vi "Process.vi"(8 "error in":errorcluster, 11 "DAQmx":refnum<class "DAQmx.lvclass">) -> (0 "error out":errorcluster, 3 "DAQmx out":refnum<class "DAQmx.lvclass">)   [LabVIEW 2019, in "DAQmx.lvclass"]
uses:
  DAQmx.lvclass
  C:/Program Files/National Instruments/LabVIEW 2019/vi.lib/JKI/JKI SMO/SMO/SMO.lvclass
  typedefs/DAQmx.Status--enum.ctl
  typedefs/DAQmx.Commands--enum.ctl
  <vilib>/JKI/JKI SMO/SMO/SMO.lvclass/SMO.ctl
  DAQmx.lvclass/DAQmx.ctl
  typedefs/Message--Cluster.ctl
  typedefs/DAQ.Config.Timing--Cluster.ctl
  typedefs/DAQ.Config.Timing.Sampling--Cluster.ctl
  typedefs/DAQ.Config.Timing.Fs Mode--enum.ctl
  <userlib>/LevyLab/Debug/Attribute.Debug/DebugBehavior.ctl
  45607b6f-cbbd-4354-99c2-ae126d9fef0d.vi
  <vilib>/JKI/JKI SMO/SMO/Private/ReftoDVR--SMO.vi
  <vilib>/JKI/JKI SMO/SMO/SMO.lvclass
  <userlib>/LevyLab/Debug/Debug.lvlib
  <userlib>/LevyLab/Debug/Attribute.Debug/Attribute.Debug.lvclass
panel:
  out "Error":string
  out "event loop":i32
  out "acq loop":i32
  out "Command":T1
  out "Status":T2
  out "State":string
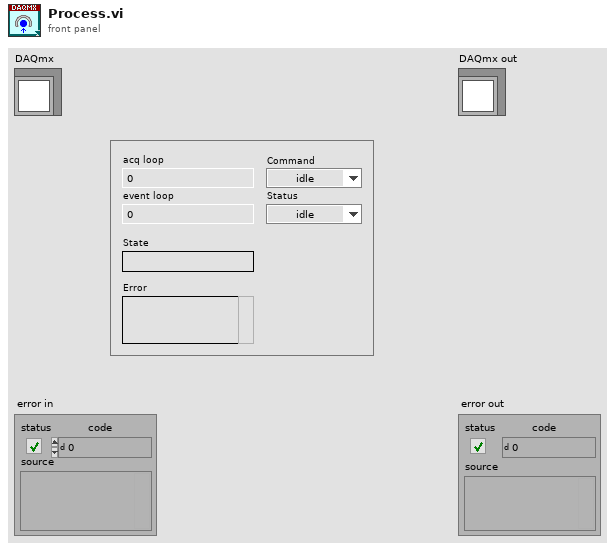
[diagram p1: front panel]
types:
  T1 = typedef "DAQmx.lvclass/DAQmx.Commands--enum.ctl" = enum16{"idle", "start", "stop", "calibrate", "auto", "exit"}
  T2 = typedef "DAQmx.lvclass/DAQmx.Status--enum.ctl" = enum16{"idle", "calibrating", "configuring", "creating", "created", "starting", "started", "stopping", "stopped", "clearing", "error"}
  T3 = typedef "Debug.lvlib/Attribute.Debug.lvclass/DebugBehavior.ctl" = enum16{"Normal", "Debug"}
  T4 = enum32{"Invalid", "Standard", "Closed", "Hidden", "Minimized", "Maximized"}
  T5 = typedef "DAQmx.lvclass/Message--Cluster.ctl" = cluster{"command":T1, "Argument":string}
  T6 = typedef "DAQmx.lvclass/DAQ.Config.Timing--Cluster.ctl" = cluster{"Sampling":T7, "sample mode":i32, "FsMode":T8, "Fs Multiplier":dbl, "Refresh Rate (Hz)":dbl, "Decimation.PreDSP":i32, "Decimation.PostDSP":i32, "Fs.Output":dbl}
  T7 = typedef "DAQmx.lvclass/DAQ.Config.Timing.Sampling--Cluster.ctl" = cluster{"Fs":dbl, "#s":i32}
  T8 = typedef "DAQmx.lvclass/DAQ.Config.Timing.Fs Mode--enum.ctl" = enum16{"Manual", "Auto Fs", "Max Fs"}
  T9 = typedef "SMO.lvclass/Protected Events.ctl" = cluster{"StopProcesses":refnum<user-event>, "AbortProcesses":refnum<user-event>, "Config Changed":refnum<user-event>, "Dependency":refnum<user-event>}
  T10 = typedef "DAQmx.lvclass/PrivateEvents--Cluster.ctl" = cluster{"Message":refnum<user-event>, "AOconfig":refnum<user-event>, "AIconfig":refnum<user-event>, "Timing":refnum<user-event>}
  T11 = cluster{"Active Device":string, "SelfCal.LastDate/Time":string, "SelfCal.LastTemp":dbl, "DevTemp":dbl, "calibration due?":bool}[]
  T12 = typedef "DAQmx.lvclass/DeviceInfo--Cluster.ctl" = cluster{"DeviceName":string, "DevIsSimulated":bool, "DeviceSerialNumber":string, "ProductType":string, "ProductCategory":i32, "ProductNumber":u32, "ChassisNumber":u32, "SlotNumber":u32, "ChassisName":string, "ChassisSerialNumber":string, "DevTemp":dbl, "SelfCal.LastDate/Time":string, "SelfCal.LastTemp":dbl, "calibration due?":bool}
  T13 = typedef "DAQmx.lvclass/DAQ.Config.AI--Cluster--Array.ctl" = T14[]
  T14 = typedef "DAQmx.lvclass/DAQ.Config.AI--Cluster.ctl" = cluster{"Channels":tag, "Coupling":T15, "Range":T16, "input terminal configuration":i32, "Type":T17}
  T15 = typedef "DAQmx.lvclass/DAQ.Config.AI.Coupling--enum.ctl" = u16
  T16 = typedef "DAQmx.lvclass/DAQ.Config.AI.Range--enum.ctl" = enum16{"±0.316", "±1.00", "±3.16", "±10.0", "±31.6", "±42.4", ""}
  T17 = typedef "DAQmx.lvclass/DAQ.Config.Device Type--enum.ctl" = enum16{"None", "USB-4431", "PXI-446x"}
  T18 = typedef "DAQmx.lvclass/DAQ.Config.AO--Cluster--Array.ctl" = T19[]
  T19 = typedef "DAQmx.lvclass/DAQ.Config.AO--Cluster.ctl" = cluster{"Channels":tag, "Range":T20, "output terminal configuration":i32, "Type":T17}
  T20 = typedef "DAQmx.lvclass/DAQ.Config.AO.Range--enum.ctl" = enum16{"±0.1", "±1.0", "±3.5", "±10.0", ""}
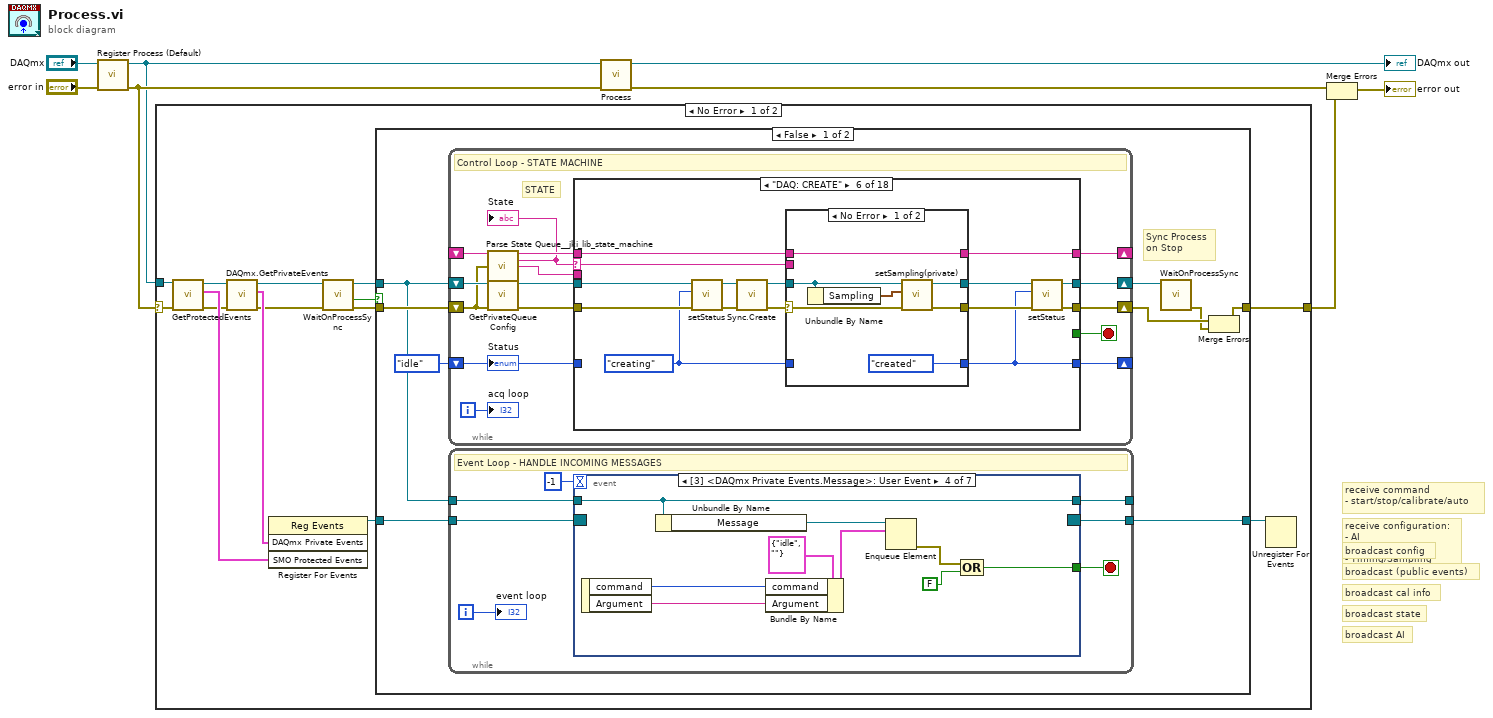
[diagram p0: block diagram]
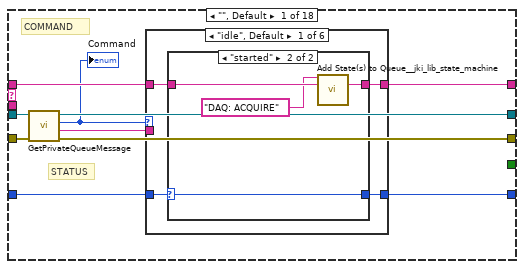
[diagram p2: hidden frame]
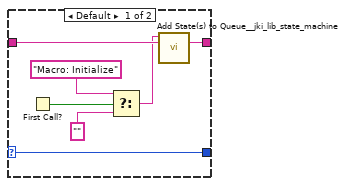
[diagram p3: hidden frame]
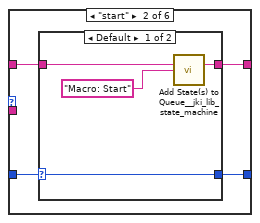
[diagram p4: hidden frame]
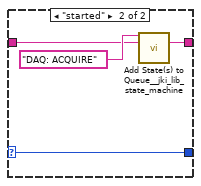
[diagram p5: hidden frame]
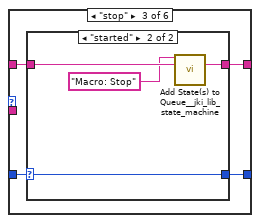
[diagram p6: hidden frame]
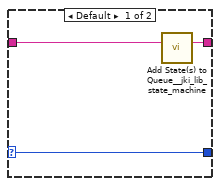
[diagram p7: hidden frame]
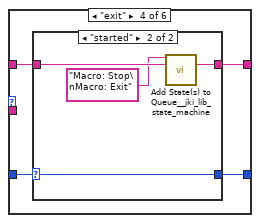
[diagram p8: hidden frame]
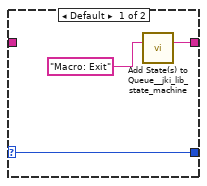
[diagram p9: hidden frame]
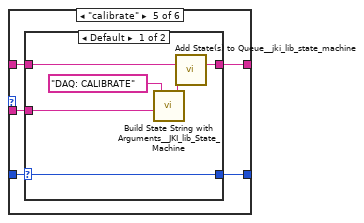
[diagram p10: hidden frame]
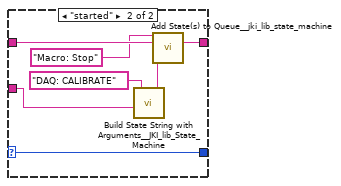
[diagram p11: hidden frame]
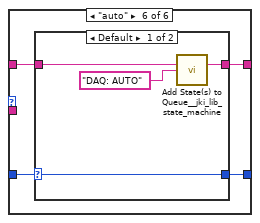
[diagram p12: hidden frame]
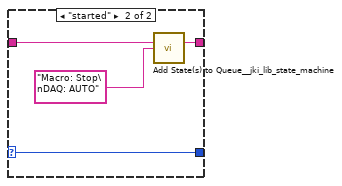
[diagram p13: hidden frame]
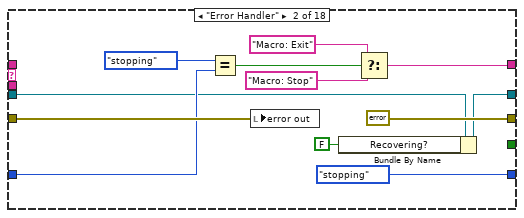
[diagram p14: hidden frame]
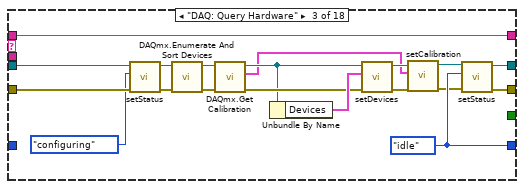
[diagram p15: hidden frame]
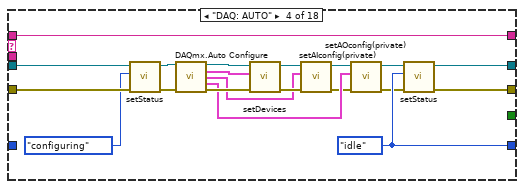
[diagram p16: hidden frame]
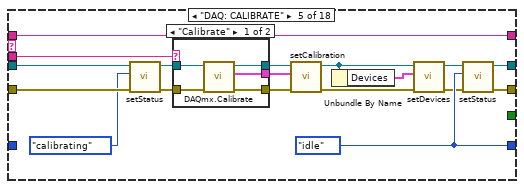
[diagram p17: hidden frame]
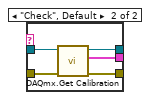
[diagram p18: hidden frame]
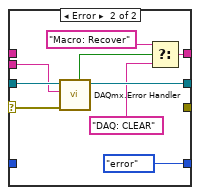
[diagram p19: hidden frame]
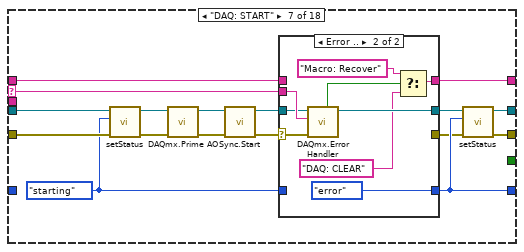
[diagram p20: hidden frame]
diagram:
  # "broadcast (public events)"
  # "receive configuration:\n- AI\n- AO\n- Timing/Sampling"
  # "receive command\n- start/stop/calibrate/auto"
  # "broadcast AI"
  # "broadcast state"
  # "broadcast cal info"
  # "broadcast config"
  n1 = call <vilib>:"Register Process (Default).vi"("error in (no error)"="error in", "SMO"="DAQmx") -> ("error out"=w3:errorcluster, "SelfRef"=w1:refnum<class "DAQmx.lvclass">)  [unwired: 8 in]
  n2 = case shown="No Error" w3 {
    selector: w3 -> [w20 w555]
    tunnel: w1 -> [w21 _]
    tunnel: [w16 w555] -> w8
    frame No Error {
      n3 = call <vilib>:"GetProtectedEvents.vi"("error in (no error)"=w20, "SMO"=w21) -> ("error out"=w13:errorcluster, "SMO Protected Events"=w22:T9, "SMO out"=w12:refnum<class "DAQmx.lvclass">)  [unwired: 7 in]
      n4 = call "DAQmx.GetPrivateEvents.vi"("error in (no error)"=w13, "DAQmx"=w12) -> ("error out"=w9:errorcluster, "DAQmx Private Events"=w11:T10, "DAQmx out"=w10:refnum<class "DAQmx.lvclass">)  [unwired: 7 in]
      n5 = register-events(w11, w22) -> (reference out=w14:refnum<event-registration>)  [unwired: 2 in, 1 out]
      n6 = call <vilib>:"WaitOnProcessSync.vi"("error in (no error)"=w9, "SMO"=w10) -> ("error out"=w18:errorcluster, "Don't run?"=w17:bool, "SMO out"=w19:refnum<class "DAQmx.lvclass">)  [unwired: 7 in]
      n7 = case shown="False" w17 {
        tunnel: w18 -> [w28 w553]
        tunnel: w19 -> [w23 _]
        tunnel: w14 -> [w30 w554]
        tunnel: [w25 w553] -> w16
        tunnel: [w29 w554] -> w15
        frame False {
          # "Sync Process\non Stop"
          n8 = while {
            shift-right: [w44] -> w31
            shift-left: w23 -> [w39]
            shift-right: [w36] -> w27
            shift-left: w28 -> [w33]
            shift-right: [w43] -> _
            shift-left: _ -> [w46]
            shift-right: [w45] -> _
            shift-left: DAQmx.Status--enum."idle" ("Status") -> [w40]
            i -> [w34]
            stop <- w32 stop-if-true
            # "STATE"
            # "Control Loop - STATE MACHINE"
            n9 = call <vilib>:"Parse State Queue__jki_lib_state_machine.vi"("State Queue"=w46, "Error In (no error)"=w33) -> ("Remaining States"=w42:string, "Current State"=w41:string, "Arguments"=w35:string)  [unwired: 11 in]
            "State" <- w41
            n10 = call "GetPrivateQueueConfig.vi"("error in (no error)"=w33, "DAQmx"=w39) -> ("error out"=w37:errorcluster, "DAQmx out"=w38:refnum<class "DAQmx.lvclass">)  [unwired: 8 in]
            n11 = case shown="\"DAQ: CREATE\"" w41 {
              selector: w41 -> [_ _ _ _ _ w222 w252 w287 w325 w348 _ _ _ _ _ _ _ _]
              tunnel: w38 -> [w51 w137 w158 w180 w202 w228 w261 w293 w330 w353 w368 w371 w377 w391 w401 w421 w431 w495]
              tunnel: [w52 w136 w159 w175 w195 w216 w248 w284 w323 w344 w368 w371 w378 w392 w399 w415 w431 w497] -> w44
              tunnel: [w49 errorcluster {"status"=FALSE, "code"=0, "source"=""} ("error out") w160 w174 w196 w215 w247 w285 w322 w345 w367 w372 w381 w390 w398 w424 _ w496] -> w36
              tunnel: w37 -> [w50 w141 w163 w179 w201 w229 w260 w292 w331 w357 w367 w372 w381 w389 w400 w420 _ w494]
              tunnel: w35 -> [_ _ _ _ w204 _ _ _ _ _ _ _ _ _ _ _ w428 _]
              tunnel: w42 -> [w53 _ w166 w186 w194 w220 w253 w290 w326 w350 _ w374 w383 w393 w409 w423 w430 w493]
              tunnel: [w56 w139 w166 w186 w194 w221 w254 w291 w327 w349 "UI: Initialize\nDAQ: Query Hardware" ("States Out") w375 w384 w394 w410 w427 w430 w493] -> w43
              tunnel: [w54 DAQmx.Status--enum."stopping" ("Status") w161 w178 w197 w217 w251 w286 w320 w343 w366 w370 w380 w395 w408 w426 w432 w499] -> w45
              tunnel: w40 -> [w55 w140 _ _ _ _ _ w289 _ _ w366 w370 w380 w395 w408 w426 w432 w499]
              tunnel: [_ _ _ _ _ _ _ _ _ _ _ _ _ _ _ _ _ TRUE] -> w32
              frame "", Default {
                # "STATUS"
                # "COMMAND"
                n12 = call "GetPrivateQueueMessage.vi"("error in (no error)"=w50, "DAQmx"=w51) -> ("error out"=w49:errorcluster, "argument"=w47:string, "command"=w48:T1, "DAQmx out"=w52:refnum<class "DAQmx.lvclass">)  [unwired: 6 in]
                "Command" <- w48
                n13 = case shown="\"idle\", Default" w48 {
                  tunnel: w55 -> [w60 w75 w87 w98 w110 w127]
                  tunnel: [w58 w74 w86 w97 w109 w126] -> w56
                  tunnel: [w59 w73 w85 w96 w108 w125] -> w54
                  tunnel: w53 -> [w57 w72 w84 w95 w107 w124]
                  tunnel: w47 -> [_ _ _ _ w106 _]
                  frame "idle", Default {
                    n14 = case shown="\"started\"" w60 {
                      selector: w60 -> [w67 w71]
                      tunnel: [w63 w69] -> w58
                      tunnel: [w67 w71] -> w59
                      tunnel: w57 -> [w62 w70]
                      frame Default {
                        n15 = First Call?() -> (First Call?: T/F=w65:bool)
                        n16 = Select(t="Macro: Initialize" ("States Out"), s=w65, f="" ("States Out")) -> (s? t:f=w61:string)
                        n17 = call <vilib>:"Add State(s) to Queue__jki_lib_state_machine.vi"("State(s) in Front (\"\")"=w61, "State(s) in (\"\")"=w62) -> ("States Out"=w63:string)  [unwired: 13 in]
                      }
                      frame "started" {
                        n18 = call <vilib>:"Add State(s) to Queue__jki_lib_state_machine.vi"("State(s) in Front (\"\")"="DAQ: ACQUIRE" ("State(s) in (\"\")"), "State(s) in (\"\")"=w70) -> ("States Out"=w69:string)  [unwired: 13 in]
                      }
                    }
                  }
                  frame "start" {
                    n19 = case shown="Default" w75 {
                      selector: w75 -> [w79 w83]
                      tunnel: [w77 w82] -> w74
                      tunnel: [w79 w83] -> w73
                      tunnel: w72 -> [w78 w80]
                      frame Default {
                        n20 = call <vilib>:"Add State(s) to Queue__jki_lib_state_machine.vi"("State(s) in (\"\")"=w78, "State(s) at Back (\"\")"="Macro: Start" ("State(s) in (\"\")")) -> ("States Out"=w77:string)  [unwired: 13 in]
                      }
                      frame "started" {
                        n21 = call <vilib>:"Add State(s) to Queue__jki_lib_state_machine.vi"("State(s) in Front (\"\")"="DAQ: ACQUIRE" ("State(s) in (\"\")"), "State(s) in (\"\")"=w80) -> ("States Out"=w82:string)  [unwired: 13 in]
                      }
                    }
                  }
                  frame "stop" {
                    n22 = case shown="\"started\"" w87 {
                      selector: w87 -> [w90 w94]
                      tunnel: [w88 w92] -> w86
                      tunnel: [w90 w94] -> w85
                      tunnel: w84 -> [w89 w93]
                      frame Default {
                        n23 = call <vilib>:"Add State(s) to Queue__jki_lib_state_machine.vi"("State(s) in (\"\")"=w89) -> ("States Out"=w88:string)  [unwired: 14 in]
                      }
                      frame "started" {
                        n24 = call <vilib>:"Add State(s) to Queue__jki_lib_state_machine.vi"("State(s) in Front (\"\")"="Macro: Stop" ("State(s) in (\"\")"), "State(s) in (\"\")"=w93) -> ("States Out"=w92:string)  [unwired: 13 in]
                      }
                    }
                  }
                  frame "exit" {
                    n25 = case shown="\"started\"" w98 {
                      selector: w98 -> [w101 w105]
                      tunnel: [w100 w102] -> w97
                      tunnel: [w101 w105] -> w96
                      tunnel: w95 -> [_ w104]
                      frame Default {
                        n26 = call <vilib>:"Add State(s) to Queue__jki_lib_state_machine.vi"("State(s) in (\"\")"="Macro: Exit" ("State(s) in (\"\")")) -> ("States Out"=w100:string)  [unwired: 14 in]
                      }
                      frame "started" {
                        n27 = call <vilib>:"Add State(s) to Queue__jki_lib_state_machine.vi"("State(s) in Front (\"\")"="Macro: Stop\nMacro: Exit" ("State(s) in (\"\")"), "State(s) in (\"\")"=w104) -> ("States Out"=w102:string)  [unwired: 13 in]
                      }
                    }
                  }
                  frame "calibrate" {
                    n28 = case shown="Default" w110 {
                      selector: w110 -> [w116 w123]
                      tunnel: [w114 w121] -> w109
                      tunnel: [w116 w123] -> w108
                      tunnel: w107 -> [w115 w122]
                      tunnel: w106 -> [w113 w119]
                      frame Default {
                        n29 = call <vilib>:"Build State String with Arguments__JKI_lib_State_Machine.vi"("Arguments (\"\")"=w113, "State"="DAQ: CALIBRATE" ("State(s) in (\"\")")) -> ("State with Arguments"=w111:string)  [unwired: 4 in]
                        n30 = call <vilib>:"Add State(s) to Queue__jki_lib_state_machine.vi"("State(s) in (\"\")"=w115, "State(s) at Back (\"\")"=w111) -> ("States Out"=w114:string)  [unwired: 13 in]
                      }
                      frame "started" {
                        n31 = call <vilib>:"Build State String with Arguments__JKI_lib_State_Machine.vi"("Arguments (\"\")"=w119, "State"="DAQ: CALIBRATE" ("State(s) in (\"\")")) -> ("State with Arguments"=w117:string)  [unwired: 4 in]
                        n32 = call <vilib>:"Add State(s) to Queue__jki_lib_state_machine.vi"("State(s) in Front (\"\")"="Macro: Stop" ("State(s) in (\"\")"), "State(s) in (\"\")"=w122, "State(s) at Back (\"\")"=w117) -> ("States Out"=w121:string)  [unwired: 12 in]
                      }
                    }
                  }
                  frame "auto" {
                    n33 = case shown="Default" w127 {
                      selector: w127 -> [w131 w135]
                      tunnel: [w129 w133] -> w126
                      tunnel: [w131 w135] -> w125
                      tunnel: w124 -> [w130 w134]
                      frame Default {
                        n34 = call <vilib>:"Add State(s) to Queue__jki_lib_state_machine.vi"("State(s) in (\"\")"=w130, "State(s) at Back (\"\")"="DAQ: AUTO" ("State(s) in (\"\")")) -> ("States Out"=w129:string)  [unwired: 13 in]
                      }
                      frame "started" {
                        n35 = call <vilib>:"Add State(s) to Queue__jki_lib_state_machine.vi"("State(s) in (\"\")"=w134, "State(s) at Back (\"\")"="Macro: Stop\nDAQ: AUTO" ("State(s) in (\"\")")) -> ("States Out"=w133:string)  [unwired: 13 in]
                      }
                    }
                  }
                }
              }
              frame "Error Handler" {
                n36 = Equal?(x=DAQmx.Status--enum."stopping" ("Status"), y=w140) -> (x = y?=w143:bool)
                n37 = local write "error out"(w141) -> ()
                n38 = Bundle By Name(cluster=w137, "Recovering?"=FALSE ("Recovery.Recovering?")) -> (w136:refnum<class "DAQmx.lvclass">)
                n39 = Select(t="Macro: Exit", s=w143, f="Macro: Stop" ("States Out")) -> (s? t:f=w139:string)
              }
              frame "DAQ: Query Hardware" {
                w161 = DAQmx.Status--enum."idle" ("setStatus")
                n40 = call "setStatus.vi"("error in (no error)"=w163, "Status"=DAQmx.Status--enum."configuring" ("setStatus"), "DAQmx in"=w158) -> ("error out"=w164:errorcluster, "DAQmx out"=w165:refnum<class "DAQmx.lvclass">)  [unwired: 7 in]
                n41 = call "DAQmx.Enumerate And Sort Devices.vi"("error in (no error)"=w164, "DAQmx in"=w165) -> ("error out"=w157:errorcluster, "DAQmx out"=w156:refnum<class "DAQmx.lvclass">)  [unwired: 7 in, 1 out]
                n42 = call "DAQmx.Get Calibration.vi"("error in (no error)"=w157, "DAQmx in"=w156) -> ("error out"=w154:errorcluster, "Calibration out"=w148:T11, "DAQmx out"=w153:refnum<class "DAQmx.lvclass">)  [unwired: 7 in]
                n43 = Unbundle By Name(w153) -> ("Devices"=w155:T12[])
                n44 = call "setDevices.vi"("error in (no error)"=w154, "Devices"=w155, "DAQmx in"=w153) -> ("error out"=w152:errorcluster, "DAQmx out"=w151:refnum<class "DAQmx.lvclass">)  [unwired: 7 in]
                n45 = call "setCalibration.vi"("error in (no error)"=w152, "Calibration out"=w148, "DAQmx in"=w151) -> ("error out"=w149:errorcluster, "DAQmx out"=w150:refnum<class "DAQmx.lvclass">)  [unwired: 7 in]
                n46 = call "setStatus.vi"("error in (no error)"=w149, "Status"=w161, "DAQmx in"=w150) -> ("error out"=w160:errorcluster, "DAQmx out"=w159:refnum<class "DAQmx.lvclass">)  [unwired: 7 in]
              }
              frame "DAQ: AUTO" {
                w178 = DAQmx.Status--enum."idle" ("setStatus")
                n47 = call "setStatus.vi"("error in (no error)"=w179, "Status"=DAQmx.Status--enum."configuring" ("setStatus"), "DAQmx in"=w180) -> ("error out"=w182:errorcluster, "DAQmx out"=w181:refnum<class "DAQmx.lvclass">)  [unwired: 7 in]
                n48 = call "DAQmx.Auto Configure.vi"("DAQmx in"=w181, "error in (no error)"=w182) -> ("DAQmx out"=w184:refnum<class "DAQmx.lvclass">, "Devices"=w167:T12[], "Configuration.AI"=w169:T13, "Configuration.AO"=w177:T18, "error out"=w185:errorcluster)  [unwired: 9 in]
                n49 = call "setDevices.vi"("error in (no error)"=w185, "Devices"=w167, "DAQmx in"=w184) -> ("error out"=w183:errorcluster, "DAQmx out"=w176:refnum<class "DAQmx.lvclass">)  [unwired: 7 in]
                n50 = call "setAIconfig(private).vi"("error in (no error)"=w183, "AIconfig"=w169, "DAQmx in"=w176) -> ("error out"=w172:errorcluster, "DAQmx out"=w173:refnum<class "DAQmx.lvclass">)  [unwired: 7 in]
                n51 = call "setAOconfig(private).vi"("error in (no error)"=w172, "AOconfig"=w177, "DAQmx in"=w173) -> ("error out"=w170:errorcluster, "DAQmx out"=w171:refnum<class "DAQmx.lvclass">)  [unwired: 7 in]
                n52 = call "setStatus.vi"("error in (no error)"=w170, "Status"=w178, "DAQmx in"=w171) -> ("error out"=w174:errorcluster, "DAQmx out"=w175:refnum<class "DAQmx.lvclass">)  [unwired: 7 in]
              }
              frame "DAQ: CALIBRATE" {
                w197 = DAQmx.Status--enum."idle" ("Status")
                n53 = call "setStatus.vi"("error in (no error)"=w201, "Status"=DAQmx.Status--enum."calibrating" ("setStatus"), "DAQmx in"=w202) -> ("error out"=w199:errorcluster, "DAQmx out"=w198:refnum<class "DAQmx.lvclass">)  [unwired: 7 in]
                n54 = case shown="\"Calibrate\"" w204 {
                  tunnel: w198 -> [w209 w214]
                  tunnel: [w208 w213] -> w188
                  tunnel: [w206 w212] -> w203
                  tunnel: w199 -> [w207 w211]
                  tunnel: [w205 w210] -> w193
                  frame "Calibrate" {
                    n55 = call "DAQmx.Calibrate.vi"("error in (no error)"=w207, "DAQmx in"=w209) -> ("error out"=w206:errorcluster, "Calibration out"=w205:T11, "DAQmx out"=w208:refnum<class "DAQmx.lvclass">)  [unwired: 7 in]
                  }
                  frame "Check", Default {
                    n56 = call "DAQmx.Get Calibration.vi"("error in (no error)"=w211, "DAQmx in"=w214) -> ("error out"=w212:errorcluster, "Calibration out"=w210:T11, "DAQmx out"=w213:refnum<class "DAQmx.lvclass">)  [unwired: 7 in]
                  }
                }
                n57 = call "setCalibration.vi"("error in (no error)"=w203, "Calibration out"=w193, "DAQmx in"=w188) -> ("error out"=w191:errorcluster, "DAQmx out"=w187:refnum<class "DAQmx.lvclass">)  [unwired: 7 in]
                n58 = Unbundle By Name(w187) -> ("Devices"=w192:T12[])
                n59 = call "setDevices.vi"("error in (no error)"=w191, "Devices"=w192, "DAQmx in"=w187) -> ("error out"=w189:errorcluster, "DAQmx out"=w190:refnum<class "DAQmx.lvclass">)  [unwired: 7 in]
                n60 = call "setStatus.vi"("error in (no error)"=w189, "Status"=w197, "DAQmx in"=w190) -> ("error out"=w196:errorcluster, "DAQmx out"=w195:refnum<class "DAQmx.lvclass">)  [unwired: 7 in]
              }
              frame "DAQ: CREATE" {
                w223 = DAQmx.Status--enum."creating" ("Status")
                n61 = call "setStatus.vi"("error in (no error)"=w229, "Status"=w223, "DAQmx in"=w228) -> ("error out"=w226:errorcluster, "DAQmx out"=w227:refnum<class "DAQmx.lvclass">)  [unwired: 7 in]
                n62 = call "Sync.Create.vi"("error in"=w226, "DAQmx in"=w227) -> ("error out"=w224:errorcluster, "DAQmx out"=w225:refnum<class "DAQmx.lvclass">)  [unwired: 8 in]
                n63 = case shown="No Error" w224 {
                  selector: w224 -> [w234 w244]
                  tunnel: w225 -> [w231 w245]
                  tunnel: [w233 _] -> w218
                  tunnel: [w232 w242] -> w219
                  tunnel: [DAQmx.Status--enum."created" ("Status") DAQmx.Status--enum."error" ("Status")] -> w217
                  tunnel: w223 -> [_ _]
                  tunnel: w222 -> [_ w241]
                  tunnel: [w236 w237] -> w221
                  tunnel: w220 -> [w236 _]
                  frame No Error {
                    n64 = Unbundle By Name(w231) -> ("Sampling"=w230:T7)
                    n65 = call "setSampling(private).vi"("error in (no error)"=w234, "Sampling"=w230, "DAQmx in"=w231) -> ("error out"=w233:errorcluster, "DAQmx out"=w232:refnum<class "DAQmx.lvclass">)  [unwired: 7 in]
                  }
                  frame Error {
                    n66 = call "DAQmx.Error Handler.vi"("error in (no error)"=w244, "[error source] (\" \")"=w241, "DAQmx in"=w245) -> ("DAQmx out"=w242:refnum<class "DAQmx.lvclass">, "retry?"=w240:bool)  [unwired: 4 in, 3 out]
                    n67 = Select(t="Macro: Recover", s=w240, f="DAQ: CLEAR" ("t")) -> (s? t:f=w237:string)
                  }
                }
                n68 = call "setStatus.vi"("error in (no error)"=w218, "Status"=w217, "DAQmx in"=w219) -> ("error out"=w215:errorcluster, "DAQmx out"=w216:refnum<class "DAQmx.lvclass">)  [unwired: 7 in]
              }
              frame "DAQ: START" {
                w255 = DAQmx.Status--enum."starting" ("Status")
                n69 = call "setStatus.vi"("error in (no error)"=w260, "Status"=w255, "DAQmx in"=w261) -> ("error out"=w259:errorcluster, "DAQmx out"=w257:refnum<class "DAQmx.lvclass">)  [unwired: 7 in]
                n70 = call "DAQmx.Prime AO.vi"("error in (no error)"=w259, "DAQmx in"=w257) -> ("error out"=w258:errorcluster, "DAQmx out"=w246:refnum<class "DAQmx.lvclass">)  [unwired: 8 in]
                n71 = call "Sync.Start.vi"("error in"=w258, "DAQmx in"=w246) -> ("error out"=w256:errorcluster, "DAQmx out"=w262:refnum<class "DAQmx.lvclass">)  [unwired: 8 in]
                n72 = case shown="Error .." w256 {
                  selector: w256 -> [w263 w273]
                  tunnel: w262 -> [w264 w274]
                  tunnel: [w263 _] -> w249
                  tunnel: [w264 w272] -> w250
                  tunnel: [DAQmx.Status--enum."started" ("Status") DAQmx.Status--enum."error" ("Status")] -> w251
                  tunnel: w255 -> [_ _]
                  tunnel: [w266 w270] -> w254
                  tunnel: w253 -> [w266 _]
                  tunnel: w252 -> [_ w275]
                  frame No Error {
                  }
                  frame Error {
                    n73 = call "DAQmx.Error Handler.vi"("error in (no error)"=w273, "[error source] (\" \")"=w275, "DAQmx in"=w274) -> ("DAQmx out"=w272:refnum<class "DAQmx.lvclass">, "retry?"=w269:bool)  [unwired: 4 in, 3 out]
                    n74 = Select(t="Macro: Recover", s=w269, f="DAQ: CLEAR" ("t")) -> (s? t:f=w270:string)
                  }
                }
                n75 = call "setStatus.vi"("error in (no error)"=w249, "Status"=w251, "DAQmx in"=w250) -> ("error out"=w247:errorcluster, "DAQmx out"=w248:refnum<class "DAQmx.lvclass">)  [unwired: 7 in]
              }
              frame "DAQ: ACQUIRE" {
                n76 = call "getWFMQueue.vi"("error in (no error)"=w292, "wait for min buffer?"=FALSE, "DAQmx in"=w293) -> ("error out"=w282:errorcluster, "DAQmx out"=w283:refnum<class "DAQmx.lvclass">)  [unwired: 6 in, 1 out]
                n77 = call "Sync.Acquire.vi"("error in (no error)"=w282, "DAQmx in"=w283) -> ("error out"=w281:errorcluster, "DAQmx out"=w280:refnum<class "DAQmx.lvclass">)  [unwired: 8 in]
                n78 = call "setWaveforms.vi"("error in (no error)"=w281, "DAQmx in"=w280) -> ("error out"=w278:errorcluster, "DAQmx out"=w279:refnum<class "DAQmx.lvclass">)  [unwired: 8 in]
                n79 = call "Scope.vi"("error in (no error)"=w278, "DAQmx in"=w279) -> ("error out"=w277:errorcluster, "DAQmx out"=w276:refnum<class "DAQmx.lvclass">)  [unwired: 8 in]
                n80 = case shown="Error .." w277 {
                  selector: w277 -> [_ w311]
                  tunnel: [w301 w315] -> w291
                  tunnel: w276 -> [w298 w319]
                  tunnel: [w296 w317] -> w284
                  tunnel: w290 -> [w301 _]
                  tunnel: w289 -> [w300 _]
                  tunnel: w287 -> [_ w312]
                  tunnel: [w300 w313] -> w286
                  tunnel: [w295 w318] -> w285
                  frame No Error {
                    n81 = call "Is Value Changed.vim"("value"=w300) -> ("changed or first call?"=w299:bool)
                    n82 = case shown="True" w299 {
                      tunnel: w298 -> [w302 w306]
                      tunnel: [w302 w305] -> w297
                      tunnel: [_ w304] -> w294
                      tunnel: w300 -> [_ w303]
                      frame False {
                      }
                      frame True {
                        n83 = call "setStatus.vi"("Status"=w303, "DAQmx in"=w306) -> ("error out"=w304:errorcluster, "DAQmx out"=w305:refnum<class "DAQmx.lvclass">)  [unwired: 8 in]
                      }
                    }
                    n84 = call "DAQmx.Acquire Recovery.vi"("error in (no error)"=w294, "DAQmx in"=w297) -> ("error out"=w295:errorcluster, "DAQmx out"=w296:refnum<class "DAQmx.lvclass">)  [unwired: 8 in]
                  }
                  frame Error {
                    w313 = DAQmx.Status--enum."error" ("t")
                    n85 = call "DAQmx.Error Handler.vi"("error in (no error)"=w311, "[error source] (\" \")"=w312, "DAQmx in"=w319) -> ("DAQmx Error?"=w307:bool, "[error Description] (\" \")"=→"Error":string, "DAQmx out"=w310:refnum<class "DAQmx.lvclass">)  [unwired: 4 in, 2 out]
                    n86 = Bundle By Name(cluster=w310, "Recovering?"=w307) -> (w309:refnum<class "DAQmx.lvclass">)
                    n87 = Select(t="Macro: Recover", s=w307, f="Macro: Stop" ("t")) -> (s? t:f=w315:string)
                    n88 = call "setStatus.vi"("Status"=w313, "DAQmx in"=w309) -> ("error out"=w318:errorcluster, "DAQmx out"=w317:refnum<class "DAQmx.lvclass">)  [unwired: 8 in]
                  }
                }
              }
              frame "DAQ: STOP" {
                w320 = DAQmx.Status--enum."stopped" ("Status")
                n89 = call "setStatus.vi"("error in (no error)"=w331, "Status"=DAQmx.Status--enum."stopping", "DAQmx in"=w330) -> ("error out"=w333:errorcluster, "DAQmx out"=w334:refnum<class "DAQmx.lvclass">)  [unwired: 7 in]
                n90 = call "Sync.Stop.vi"("error in (no error)"=w333, "DAQmx in"=w334) -> ("error out"=w329:errorcluster, "DAQmx out"=w332:refnum<class "DAQmx.lvclass">)  [unwired: 8 in]
                n91 = case shown="Error .." w329 {
                  selector: w329 -> [w335 w341]
                  tunnel: w332 -> [w337 w339]
                  tunnel: [w337 w340] -> w324
                  tunnel: [w336 w338] -> w327
                  tunnel: w326 -> [w336 w338]
                  tunnel: w325 -> [_ w342]
                  tunnel: [w335 _] -> w321
                  frame No Error {
                  }
                  frame Error {
                    n92 = call "DAQmx.Error Handler.vi"("error in (no error)"=w341, "[error source] (\" \")"=w342, "DAQmx in"=w339) -> ("DAQmx out"=w340:refnum<class "DAQmx.lvclass">)  [unwired: 4 in, 4 out]
                  }
                }
                n93 = call "setStatus.vi"("error in (no error)"=w321, "Status"=w320, "DAQmx in"=w324) -> ("error out"=w322:errorcluster, "DAQmx out"=w323:refnum<class "DAQmx.lvclass">)  [unwired: 7 in]
              }
              frame "DAQ: CLEAR" {
                w343 = DAQmx.Status--enum."idle" ("Status")
                n94 = call "setStatus.vi"("error in (no error)"=w357, "Status"=DAQmx.Status--enum."clearing", "DAQmx in"=w353) -> ("error out"=w355:errorcluster, "DAQmx out"=w356:refnum<class "DAQmx.lvclass">)  [unwired: 7 in]
                n95 = call "Sync.Destroy.vi"("error in (no error)"=w355, "DAQmx in"=w356) -> ("error out"=w351:errorcluster, "DAQmx out"=w354:refnum<class "DAQmx.lvclass">)  [unwired: 8 in]
                n96 = case shown="Error .." w351 {
                  selector: w351 -> [w359 w363]
                  tunnel: w354 -> [w360 w364]
                  tunnel: [w360 w362] -> w347
                  tunnel: [w359 _] -> w346
                  tunnel: w350 -> [w358 w361]
                  tunnel: [w358 w361] -> w349
                  tunnel: w348 -> [_ w365]
                  frame No Error {
                  }
                  frame Error {
                    n97 = call "DAQmx.Error Handler.vi"("error in (no error)"=w363, "[error source] (\" \")"=w365, "DAQmx in"=w364) -> ("DAQmx out"=w362:refnum<class "DAQmx.lvclass">)  [unwired: 4 in, 4 out]
                  }
                }
                n98 = call "setStatus.vi"("error in (no error)"=w346, "Status"=w343, "DAQmx in"=w347) -> ("error out"=w345:errorcluster, "DAQmx out"=w344:refnum<class "DAQmx.lvclass">)  [unwired: 7 in]
              }
              frame "Macro: Initialize" {
              }
              frame "Macro: Start" {
                n99 = call <vilib>:"Add State(s) to Queue__jki_lib_state_machine.vi"("State(s) in Front (\"\")"="DAQ: CREATE\nDAQ: START\nDAQ: ACQUIRE" ("State(s) in Front (\"\")"), "State(s) in (\"\")"=w374) -> ("States Out"=w375:string)  [unwired: 13 in]
              }
              frame "Macro: Stop" {
                w376 = waveform(dbl)[] [] ("Recovery.Pending AO")
                n100 = Bundle By Name(cluster=w377, "Recovering?"=FALSE ("Recovery.Recovering?"), "Pending AO"=w376, "Pending REF_X"=w376, "Pending REF_Y"=w376) -> (w378:refnum<class "DAQmx.lvclass">)
                n101 = call <vilib>:"Add State(s) to Queue__jki_lib_state_machine.vi"("State(s) in Front (\"\")"="DAQ: STOP\nDAQ: CLEAR" ("State(s) in Front (\"\")"), "State(s) in (\"\")"=w383) -> ("States Out"=w384:string)  [unwired: 13 in]
              }
              frame "Macro: Recover" {
                n102 = call "DAQmx.Recovery Error Handler.vi"("error in (no error)"=w389, "DAQmx in"=w391) -> ("error out"=w390:errorcluster, "retry?"=w388:bool, "DAQmxout"=w392:refnum<class "DAQmx.lvclass">)  [unwired: 7 in]
                n103 = Select(t="DAQ: STOP\nDAQ: CLEAR\nDAQ: CREATE\nDAQ: START\nDAQ: ACQUIRE" ("State(s) in Front (\"\")"), s=w388, f="Macro: Stop" ("State(s) in Front (\"\")")) -> (s? t:f=w386:string)
                n104 = call <vilib>:"Add State(s) to Queue__jki_lib_state_machine.vi"("State(s) in Front (\"\")"=w386, "State(s) in (\"\")"=w393) -> ("States Out"=w394:string)  [unwired: 13 in]
              }
              frame "Macro: Exit" {
                n105 = call <userlib>:"Get Debug Mode.vi"("error in (no error)"=w400, "SMO"=w401) -> ("error out"=w398:errorcluster, "Behavior"=w404:T3, "SMO out"=w399:refnum<class "DAQmx.lvclass">)  [unwired: 7 in]
                n106 = Equal?(x=DebugBehavior."Debug", y=w404) -> (x = y?=w407:bool)
                n107 = Select(t="Open", s=w407, f="Close") -> (s? t:f=w405:string)
                n108 = Format Into String(format string="UI: Front Panel State >> %s\nexit" ("State(s) in Front (\"\")"), w405) -> (resulting string=w396:string)  [unwired: 2 in, 1 out]
                n109 = call <vilib>:"Add State(s) to Queue__jki_lib_state_machine.vi"("State(s) in Front (\"\")"=w396, "State(s) in (\"\")"=w409) -> ("States Out"=w410:string)  [unwired: 13 in]
              }
              frame "UI: Initialize" {
                n110 = call <userlib>:"Get Debug Mode.vi"("error in (no error)"=w420, "SMO"=w421) -> ("error out"=w414:errorcluster, "Behavior"=w413:T3, "SMO out"=w415:refnum<class "DAQmx.lvclass">)  [unwired: 7 in]
                n111 = Equal?(x=DebugBehavior."Debug", y=w413) -> (x = y?=w422:bool)
                n112 = Select(t="Open", s=w422, f="Close") -> (s? t:f=w418:string)
                n113 = Format Into String(format string="UI: Front Panel State >> %s" ("State(s) in Front (\"\")"), w418) -> (resulting string=w416:string)  [unwired: 2 in, 1 out]
                n114 = call <userlib>:"Fit VI window to Largest Dec__ogtk.vi"("error in (no error)"=w414, "border spacing (2 px)"=0) -> ("error out"=w424:errorcluster)  [unwired: 4 in, 1 out]
                n115 = call <vilib>:"Add State(s) to Queue__jki_lib_state_machine.vi"("State(s) in Front (\"\")"=w416, "State(s) in (\"\")"=w423) -> ("States Out"=w427:string)  [unwired: 13 in]
              }
              frame "UI: Front Panel State" {
                n116 = control-ref of="Current VI Reference"() -> (w429:refnum<vi>)
                n117 = case shown="\"Minimize\", \"Minimized\"" w428 {
                  tunnel: [w439 w452 w463 w475 w487] -> _
                  tunnel: w429 -> [w438 w450 w462 w474 w486]
                  frame "Open", "Standard", Default {
                    w433 = T4."Standard" ("State")
                    n118 = property class="VI"(reference=w438) -> (reference out=w436:refnum<vi>, error out=w437:errorcluster, "FP.State"=w435:T4)  [unwired: 1 in]
                    n119 = Not Equal?(x=w435, y=w433) -> (x != y?=w434:bool)
                    n120 = case shown="True" w434 {
                      tunnel: [w443 w445] -> w439
                      tunnel: w437 -> [w442 w445]
                      tunnel: w436 -> [w441 _]
                      tunnel: w433 -> [w440 _]
                      frame True {
                        n121 = invoke class="VI" method="FP.Open"(reference=w441, error in=w442, "Activate"=TRUE, "State"=w440) -> (error out=w443:errorcluster)  [unwired: 1 in, 4 out]
                      }
                      frame False {
                      }
                    }
                  }
                  frame "Close", "Closed" {
                    n122 = property class="VI"(reference=w450) -> (reference out=w449:refnum<vi>, error out=w451:errorcluster, "FP.State"=w447:T4)  [unwired: 1 in]
                    n123 = Not Equal?(x=w447, y=T4."Closed" ("Front Panel Window:State")) -> (x != y?=w446:bool)
                    n124 = case shown="True" w446 {
                      tunnel: [w453 w456] -> w452
                      tunnel: w451 -> [w453 w455]
                      tunnel: w449 -> [_ w454]
                      frame False {
                      }
                      frame True {
                        n125 = invoke class="VI" method="FP.Close"(reference=w454, error in=w455) -> (error out=w456:errorcluster)  [unwired: 1 in, 2 out]
                      }
                    }
                  }
                  frame "Hidden", "Hide" {
                    w457 = T4."Hidden" ("State")
                    n126 = property class="VI"(reference=w462) -> (reference out=w460:refnum<vi>, error out=w461:errorcluster, "FP.State"=w459:T4)  [unwired: 1 in]
                    n127 = Not Equal?(x=w459, y=w457) -> (x != y?=w458:bool)
                    n128 = case shown="True" w458 {
                      tunnel: [w467 w468] -> w463
                      tunnel: w461 -> [w466 w468]
                      tunnel: w460 -> [w465 _]
                      tunnel: w457 -> [w464 _]
                      frame True {
                        n129 = invoke class="VI" method="FP.Open"(reference=w465, error in=w466, "State"=w464) -> (error out=w467:errorcluster)  [unwired: 2 in, 4 out]
                      }
                      frame False {
                      }
                    }
                  }
                  frame "Minimize", "Minimized" {
                    w469 = T4."Minimized" ("State")
                    n130 = property class="VI"(reference=w474) -> (reference out=w472:refnum<vi>, error out=w473:errorcluster, "FP.State"=w471:T4)  [unwired: 1 in]
                    n131 = Not Equal?(x=w471, y=w469) -> (x != y?=w470:bool)
                    n132 = case shown="True" w470 {
                      tunnel: [w479 w480] -> w475
                      tunnel: w473 -> [w478 w480]
                      tunnel: w472 -> [w477 _]
                      tunnel: w469 -> [w476 _]
                      frame True {
                        n133 = invoke class="VI" method="FP.Open"(reference=w477, error in=w478, "State"=w476) -> (error out=w479:errorcluster)  [unwired: 2 in, 4 out]
                      }
                      frame False {
                      }
                    }
                  }
                  frame "Maximize", "Maximized" {
                    w481 = T4."Maximized" ("State")
                    n134 = property class="VI"(reference=w486) -> (reference out=w484:refnum<vi>, error out=w485:errorcluster, "FP.State"=w483:T4)  [unwired: 1 in]
                    n135 = Not Equal?(x=w483, y=w481) -> (x != y?=w482:bool)
                    n136 = case shown="True" w482 {
                      tunnel: [w491 w492] -> w487
                      tunnel: w485 -> [w490 w492]
                      tunnel: w484 -> [w489 _]
                      tunnel: w481 -> [w488 _]
                      frame True {
                        n137 = invoke class="VI" method="FP.Open"(reference=w489, error in=w490, "State"=w488) -> (error out=w491:errorcluster)  [unwired: 2 in, 4 out]
                      }
                      frame False {
                      }
                    }
                  }
                }
              }
              frame "exit" {
                n138 = call <vilib>:"SelfTerminate.vi"("error in (no error)"=w494, "SMO in"=w495) -> ("error out"=w496:errorcluster, "SMO out"=w497:refnum<class "DAQmx.lvclass">)  [unwired: 8 in]
              }
            }
            "Status" <- w40
            "acq loop" <- w34
          }
          n139 = while {
            tunnel: w30 -> [w505]
            tunnel: [w504] -> w29
            tunnel: [w502] -> _
            tunnel: w23 -> [w501]
            i -> [w500]
            stop <- w503 stop-if-true
            # "Event Loop - HANDLE INCOMING MESSAGES"
            n140 = event shown="[3] <DAQmx Private Events.Message>: User Event" {
              selector: w505 -> [_ _ _ _ _ _ _]
              dyn-events: [_ _ _ _ _ _ _] -> w504
              timeout: -1 -> [_ _ _ _ _ _ _]
              tunnel: [_ TRUE TRUE w531 w538 w544 w552] -> w503
              tunnel: [w507 w514 w520 w529 w535 w542 w549] -> w502
              tunnel: w501 -> [w507 w514 w520 w529 w535 w542 w549]
              event Timeout {
                n141 = event-data() -> ()  [unwired: 1 in, 1 out]
              }
              event User Event {
                # "Stop SMO"
                n142 = event-data() -> ()  [unwired: 1 in, 1 out]
                n143 = Unbundle By Name(w514) -> ("Message"=w511:refnum<queue>)
                n144 = Bundle By Name(cluster=T5 {"command"=enum."idle", "Argument"=""} ("Message"), "command"=DAQmx.Commands--enum."exit" ("notification")) -> (w510:T5)
                n145 = Enqueue Element(queue=w511, element=w510) -> (error out=w512:errorcluster)  [unwired: 2 in, 2 out]
                n146 = Compound Arithmetic op=OR(w512, FALSE) -> ()  [unwired: 1 out]
              }
              event User Event {
                # "Abort SMO"
                n147 = event-data() -> ()  [unwired: 1 in, 1 out]
                n148 = Unbundle By Name(w520) -> ("Message"=w519:refnum<queue>)
                n149 = Bundle By Name(cluster=T5 {"command"=enum."idle", "Argument"=""} ("Message"), "command"=DAQmx.Commands--enum."exit" ("notification")) -> (w516:T5)
                n150 = Enqueue Element(queue=w519, element=w516) -> (error out=w521:errorcluster)  [unwired: 2 in, 2 out]
                n151 = Compound Arithmetic op=OR(w521, FALSE) -> ()  [unwired: 1 out]
              }
              event User Event {
                n152 = event-data() -> ("command"=w527:T1, "Argument"=w526:string)  [unwired: 1 in]
                n153 = Unbundle By Name(w529) -> ("Message"=w524:refnum<queue>)
                n154 = Bundle By Name(cluster=T5 {"command"=enum."idle", "Argument"=""} ("Message"), "command"=w527, "Argument"=w526) -> (w525:T5)
                n155 = Enqueue Element(queue=w524, element=w525) -> (error out=w530:errorcluster)  [unwired: 2 in, 2 out]
                n156 = Compound Arithmetic op=OR(w530, FALSE) -> (w531:bool)
              }
              event User Event {
                n157 = event-data() -> ("AOconfig"=w533:T18)  [unwired: 1 in]
                n158 = Unbundle By Name(w535) -> ("AOconfig"=w534:refnum<queue>)
                n159 = Enqueue Element(queue=w534, element=w533) -> (error out=w536:errorcluster)  [unwired: 2 in, 2 out]
                n160 = Compound Arithmetic op=OR(w536, FALSE) -> (w538:bool)
              }
              event User Event {
                n161 = event-data() -> ("AIconfig"=w540:T13)  [unwired: 1 in]
                n162 = Unbundle By Name(w542) -> ("AIconfig"=w539:refnum<queue>)
                n163 = Enqueue Element(queue=w539, element=w540) -> (error out=w541:errorcluster)  [unwired: 2 in, 2 out]
                n164 = Compound Arithmetic op=OR(w541, FALSE) -> (w544:bool)
              }
              event User Event {
                n165 = event-data() -> ("Sampling"=w548:T7)  [unwired: 1 in]
                n166 = Unbundle By Name(w549) -> ("Timing"=w546:refnum<queue>)
                n167 = Bundle By Name(cluster=T6 {"Sampling"={"Fs"=1000.0, "#s"=128}, "sample mode"=10123, "FsMode"=enum."Manual", "Fs Multiplier"=1.0, "Refresh Rate (Hz)"=10.0, "Decimation.PreDSP"=1, "Decimation.PostDSP"=1, "Fs.Output"=204789.0} ("Timing"), "Sampling"=w548) -> (w545:T6)
                n168 = Enqueue Element(queue=w546, element=w545) -> (error out=w547:errorcluster)  [unwired: 2 in, 2 out]
                n169 = Compound Arithmetic op=OR(w547, FALSE) -> (w552:bool)
              }
            }
            "event loop" <- w500
          }
          n170 = call <vilib>:"WaitOnProcessSync.vi"("SMO"=w31) -> ("error out"=w26:errorcluster)  [unwired: 8 in, 2 out]
          n171 = Merge Errors(w27, w26) -> (w25:errorcluster)
        }
        frame True {
        }
      }
      n172 = Unregister For Events(event registration refnum=w15) -> ()  [unwired: 1 in, 1 out]
    }
    frame Error {
    }
  }
  n173 = call-parent "Process.vi"("error in"=w3, "SMO"=w1) -> ("error out"=w7:errorcluster, "SMO out"=→"DAQmx out":refnum<class "DAQmx.lvclass">)  [unwired: 8 in]
  n174 = Merge Errors(w7, w8) -> (→"error out":errorcluster)
